vi "create.vi"(6 "be tolerant against empty path?":bool, 8 "error in (no error)":errorcluster, 10 "class path":path) -> (0 "error out":errorcluster, 3 "GenericAdapter out":refnum<class "GenericAdapter.lvclass">)   [LabVIEW 2010, in "GenericAdapter.lvclass"]
uses:
  GenericAdapter.lvclass
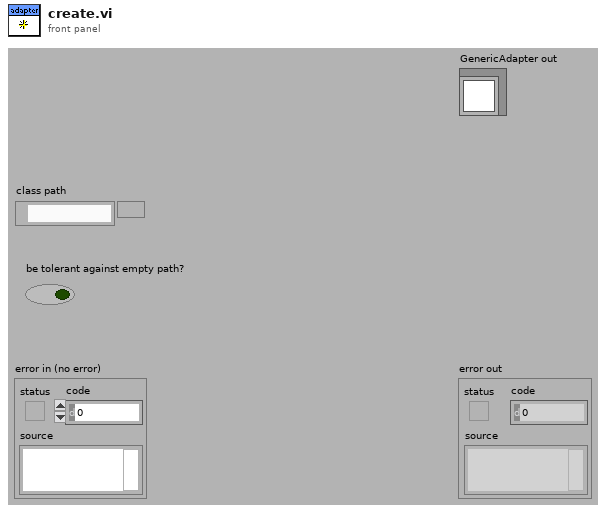
[diagram p1: front panel]
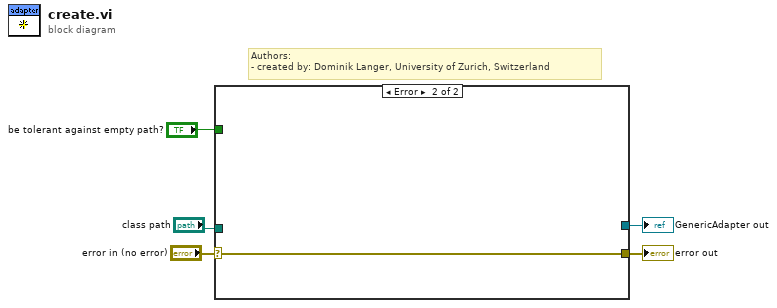
[diagram p0: block diagram]
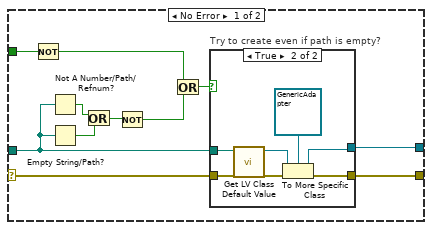
[diagram p2: hidden frame]
diagram:
  # "Authors: \n- created by: Dominik Langer, University of Zurich, Switzerland"
  n1 = case shown="Error" "error in (no error)" {
    selector: "error in (no error)" -> [w16 w25]
    tunnel: [w15 w25] -> w4
    tunnel: [w14 _] -> w3
    tunnel: "class path" -> [w12 _]
    tunnel: "be tolerant against empty path?" -> [w13 _]
    frame No Error {
      n2 = Not(x=w13) -> (.not. x?=w9:bool)
      n3 = Not A Number/Path/Refnum?(number/path/refnum=w12) -> (NaN/Path/Refnum?=w11:bool)
      n4 = Empty String/Path?(string/path=w12) -> (empty?=w10:bool)
      n5 = Or(x=w11, y=w10) -> (x .or. y?=w8:bool)
      n6 = Not(x=w8) -> (.not. x?=w7:bool)
      n7 = Or(x=w9, y=w7) -> (x .or. y?=w6:bool)
      n8 = case "Try to create even if path is empty?" shown="True" w6 {
        tunnel: w16 -> [w17 w24]
        tunnel: [w17 w22] -> w15
        tunnel: [_ w19] -> w14
        tunnel: w12 -> [_ w18]
        frame False {
        }
        frame True {
          n9 = call <vilib>:"Get LV Class Default Value.vi"("error in (no error)"=w24, "class path"=w18) -> ("error out"=w23:errorcluster, "object"=w21:refnum<class>)  [unwired: 8 in]
          n10 = To More Specific Class(target class=refnum<class "GenericAdapter.lvclass"> refnum ("GenericAdapter.lvclass"), reference=w21, error in=w23) -> (specific class reference=w19:refnum<class "GenericAdapter.lvclass">, error out=w22:errorcluster)
        }
      }
    }
    frame Error {
    }
  }
  "error out" <- w4
  "GenericAdapter out" <- w3
